vi "Get PCL Decimation_ex.vi"() -> ()   [LabVIEW 2019]
uses:
  <vilib>/NI VeriStand/Custom Device API/Custom Device Item Ref.ctl
  Scripting API/Scripting API.lvlib
  <vilib>/NI VeriStand/Custom Device API/Custom Device API.lvlib
panel:
  in  "Instrument Addon Refnum In":T1=18446744073709551615 format="%.0x"
  out "Instrument Addon Refnum Out":T1=18446744073709551615 format="%.0x"
  out "PCL Decimation":u16
  out "Error Out":errorcluster
  in  "Error In":errorcluster
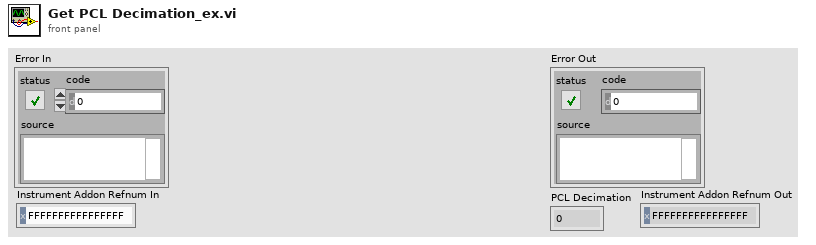
[diagram p1: front panel]
types:
  T1 = typedef "Custom Device API.lvlib/Custom Device Item Ref.ctl" = u64
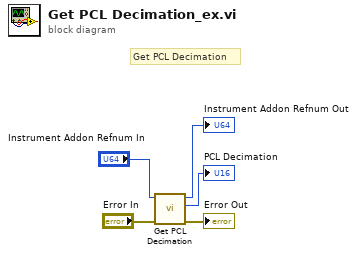
[diagram p0: block diagram]
diagram:
  # "Get PCL Decimation"
  n1 = call "Get PCL Decimation.vi"("Error In"="Error In", "Instrument Addon Refnum In"="Instrument Addon Refnum In") -> ("Error Out"=→"Error Out":errorcluster, "PCL Decimation"=→"PCL Decimation":u16, "Instrument Addon Refnum Out"=→"Instrument Addon Refnum Out":T1)  [unwired: 7 in]
